vi "zad2.vi"() -> ()   [LabVIEW 2017]
uses:
  Stan.ctl
panel:
  in  "Stan 6":bool
  in  "Stan 4":bool
  in  "Stan 5":bool
  in  "Stan 3":bool
  in  "Stan 2":bool
  in  "Stan 7":bool
  in  "Stan 1":bool
  in  "Start":bool
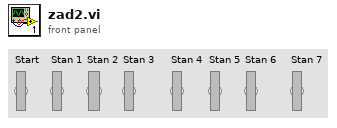
[diagram p1: front panel]
types:
  T1 = typedef "Stan.ctl" = enum16{"Start", "Stan 1", "Stan 2", "Stan 3", "Stan 4", "Stan 5", "Stan 6", "Stan 7", "Koniec"}
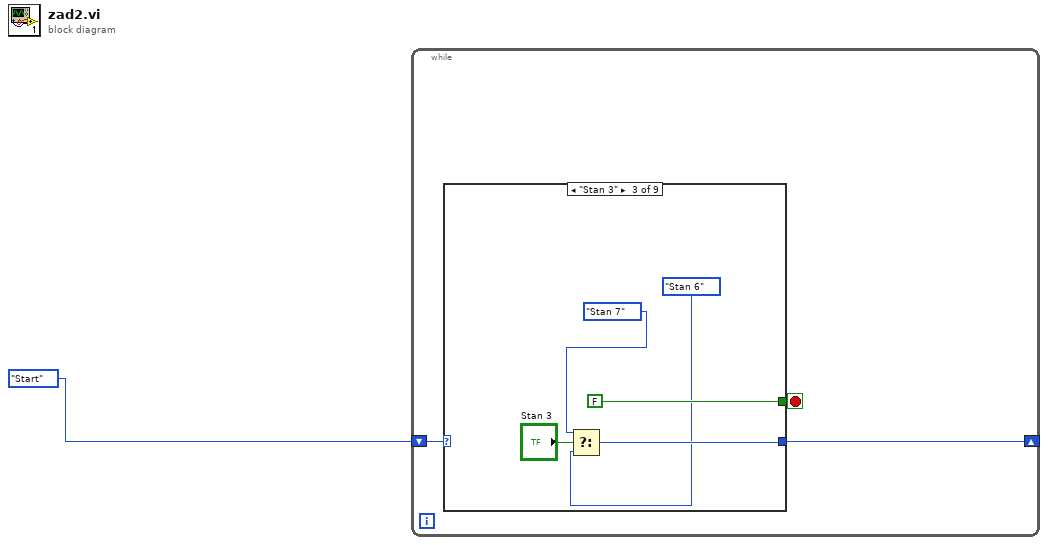
[diagram p0: block diagram]
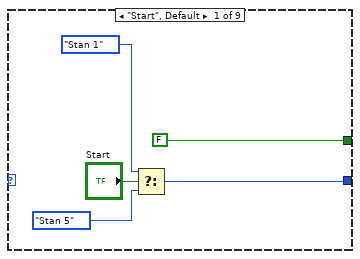
[diagram p2: hidden frame]
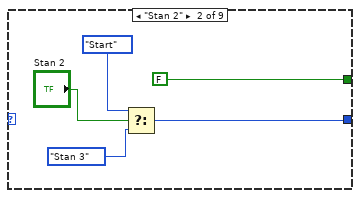
[diagram p3: hidden frame]
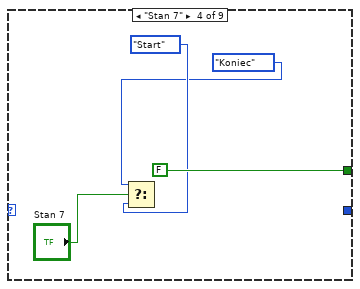
[diagram p4: hidden frame]
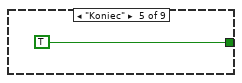
[diagram p5: hidden frame]
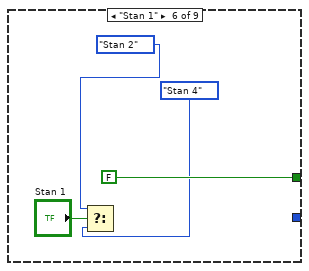
[diagram p6: hidden frame]
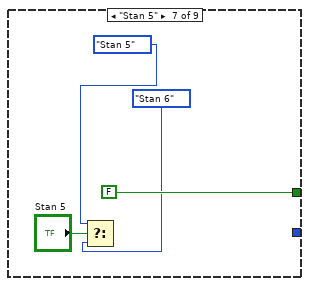
[diagram p7: hidden frame]
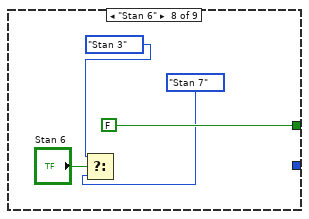
[diagram p8: hidden frame]
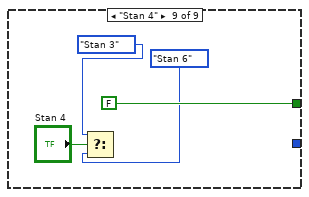
[diagram p9: hidden frame]
diagram:
  n1 = while {
    shift-right: [w2] -> _
    shift-left: Stan."Start" ("Enum") -> [w4]
    stop <- w3 stop-if-true
    n2 = case shown="\"Stan 3\"" w4 {
      tunnel: [w8 w13 w19 _ _ _ _ _ _] -> w2
      tunnel: [FALSE FALSE FALSE FALSE TRUE FALSE FALSE FALSE FALSE] -> w3
      frame "Start", Default {
        n3 = Select(t=Stan."Stan 1" ("Enum"), s="Start", f=Stan."Stan 5" ("Enum")) -> (s? t:f=w8:T1)
      }
      frame "Stan 2" {
        n4 = Select(t=Stan."Start" ("Enum"), s="Stan 2", f=Stan."Stan 3" ("Enum")) -> (s? t:f=w13:T1)
      }
      frame "Stan 3" {
        n5 = Select(t=Stan."Stan 7" ("Enum"), s="Stan 3", f=Stan."Stan 6" ("Enum")) -> (s? t:f=w19:T1)
      }
      frame "Stan 7" {
        n6 = Select(t=Stan."Koniec" ("Enum"), s="Stan 7", f=Stan."Start" ("Enum")) -> ()  [unwired: 1 out]
      }
      frame "Koniec" {
      }
      frame "Stan 1" {
        n7 = Select(t=Stan."Stan 2" ("Enum"), s="Stan 1", f=Stan."Stan 4" ("Enum")) -> ()  [unwired: 1 out]
      }
      frame "Stan 5" {
        n8 = Select(t=Stan."Stan 5" ("Enum"), s="Stan 5", f=Stan."Stan 6" ("Enum")) -> ()  [unwired: 1 out]
      }
      frame "Stan 6" {
        n9 = Select(t=Stan."Stan 3" ("Enum"), s="Stan 6", f=Stan."Stan 7" ("Enum")) -> ()  [unwired: 1 out]
      }
      frame "Stan 4" {
        n10 = Select(t=Stan."Stan 3" ("Enum"), s="Stan 4", f=Stan."Stan 6" ("Enum")) -> ()  [unwired: 1 out]
      }
    }
  }
